vi "SERIAL_DecodeStreamResponse.vi"(8 "error in":errorcluster, 10 "Buffer":string, 11 "navX DevRef":T1={"SerialPortRef"={"DevStatus"={"status"=FALSE, "code"=0, "source"=""}, "Serial Port Name"=""}, "Board Information"={"WhoAmI (50 | 0x32)"=0, "Board Revision"=0, "Firmware Major Version"=0, "Firmware Minor Version"=0}, "Status"={"Update Rate Hz"=0, "Accelerometer Full-Scale Range"=0, "Gyro Full-Scale Range"=0, "NAVX_OP_STATUS"=0, "NAVX_CAL_STATUS"=0, "NAVX_SELFTEST_STATUS"=0, "NAVX_SENSOR_STATUS"=0}, "Offsets"={"Yaw"=0.0, "Quat W"=0.0, "Quat X"=0.0, "Quat Y"=0.0, "Quat Z"=0.0}, "Update Rate (4Hz-60Hz)"=50, "Nav6Mode (YPR)"=enum."YPR", "refnum name"="", "error"={"status"=FALSE, "code"=0, "source"=""}} {"Status"."NAVX_OP_STATUS" items=["INITIALIZING", "SELFTEST_IN_PROGRESS", "ERROR", "IMU_AUTOCAL_IN_PROGRESS", "NORMAL"]; "Status"."NAVX_CAL_STATUS" items=["IMU_CAL_STATE_MASK"=3, "IMU_CAL_INPROGRESS"=0, "IMU_CAL_ACCUMULATE"=1, "IMU_CAL_COMPLETE"=2, "MAG_CAL_COMPLETE"=4, "BARO_CAL_COMPLETE"=8]}) -> (0 "error out":errorcluster, 2 "Valid":bool, 3 "navX DevRef":T1={"SerialPortRef"={"DevStatus"={"status"=FALSE, "code"=0, "source"=""}, "Serial Port Name"=""}, "Board Information"={"WhoAmI (50 | 0x32)"=0, "Board Revision"=0, "Firmware Major Version"=0, "Firmware Minor Version"=0}, "Status"={"Update Rate Hz"=0, "Accelerometer Full-Scale Range"=0, "Gyro Full-Scale Range"=0, "NAVX_OP_STATUS"=0, "NAVX_CAL_STATUS"=0, "NAVX_SELFTEST_STATUS"=0, "NAVX_SENSOR_STATUS"=0}, "Offsets"={"Yaw"=0.0, "Quat W"=0.0, "Quat X"=0.0, "Quat Y"=0.0, "Quat Z"=0.0}, "Update Rate (4Hz-60Hz)"=50, "Nav6Mode (YPR)"=enum."YPR", "refnum name"="", "error"={"status"=FALSE, "code"=0, "source"=""}} {"Status"."NAVX_OP_STATUS" items=["INITIALIZING", "SELFTEST_IN_PROGRESS", "ERROR", "IMU_AUTOCAL_IN_PROGRESS", "NORMAL"]; "Status"."NAVX_CAL_STATUS" items=["IMU_CAL_STATE_MASK"=3, "IMU_CAL_INPROGRESS"=0, "IMU_CAL_ACCUMULATE"=1, "IMU_CAL_COMPLETE"=2, "MAG_CAL_COMPLETE"=4, "BARO_CAL_COMPLETE"=8]})   [LabVIEW 2014, in "navX-MXP IMU.lvlib"]
uses:
  navX-MXP IMU.lvlib
  navX Serial DevRef.ctl
  <vilib>/Rock Robotics/WPI/SerialPort/WPI_SerialPortRef.ctl
  COMMON/TypeDefs/navX Board Information.ctl
  COMMON/TypeDefs/navX Status Data.ctl
  COMMON/TypeDefs/navX NAVX_OP_STATUS.ctl
  COMMON/TypeDefs/navX NAVX_CAL_STATUS.ctl
  TypeDefs/navX Serial Mode.ctl
  COMMON/TypeDefs/navX Offsets Data.ctl
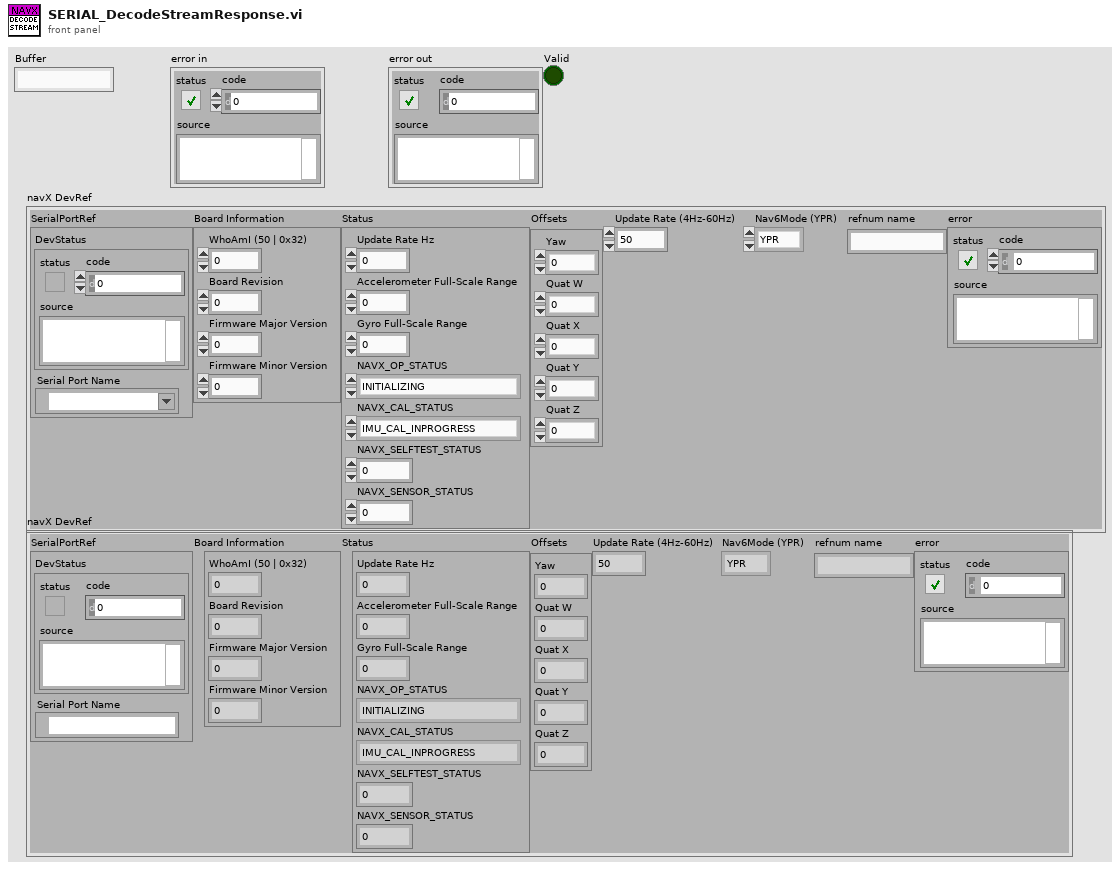
[diagram p1: front panel]
types:
  T1 = typedef "navX-MXP IMU.lvlib/navX Serial DevRef.ctl" = cluster{"SerialPortRef":T2, "Board Information":T3, "Status":T4, "Offsets":cluster{"Yaw":dbl, "Quat W":dbl, "Quat X":dbl, "Quat Y":dbl, "Quat Z":dbl}, "Update Rate (4Hz-60Hz)":u8, "Nav6Mode (YPR)":T7, "refnum name":string, "error":errorcluster}
  T2 = typedef "WPI_SerialPortRef.ctl" = cluster{"DevStatus":errorcluster, "Serial Port Name":refnum<visa-resource-name>}
  T3 = typedef "navX-MXP IMU.lvlib/navX Board Information.ctl" = cluster{"WhoAmI (50 | 0x32)":u8, "Board Revision":u8, "Firmware Major Version":u8, "Firmware Minor Version":u8}
  T4 = typedef "navX-MXP IMU.lvlib/navX Status Data.ctl" = cluster{"Update Rate Hz":u8, "Accelerometer Full-Scale Range":u8, "Gyro Full-Scale Range":u16, "NAVX_OP_STATUS":T5, "NAVX_CAL_STATUS":T6, "NAVX_SELFTEST_STATUS":u8, "NAVX_SENSOR_STATUS":u16}
  T5 = typedef "navX-MXP IMU.lvlib/navX NAVX_OP_STATUS.ctl" = u8
  T6 = typedef "navX-MXP IMU.lvlib/navX NAVX_CAL_STATUS.ctl" = u8
  T7 = typedef "navX-MXP IMU.lvlib/navX Serial Mode.ctl" = enum16{"YPR", "Gyro", "Quaternion"}
  T8 = typedef "navX-MXP IMU.lvlib/navX Offsets Data.ctl" = cluster{"Yaw":dbl, "Quat W":dbl, "Quat X":dbl, "Quat Y":dbl, "Quat Z":dbl}
  T9 = cluster{"Gyroscope Full Scale Range":u32, "Accelerometer Full Scale Range":u32, "Update Rate":u32, "Calibrated Yaw Offset":dbl, "Calibrated Quaternion W Offset ":u32, "Calibrated Quaternion X Offset":u32, "Calibrated Quaternion Y Offset":u32, "Calibrated Quaternion Z Offset":u32, "Flags":u32}
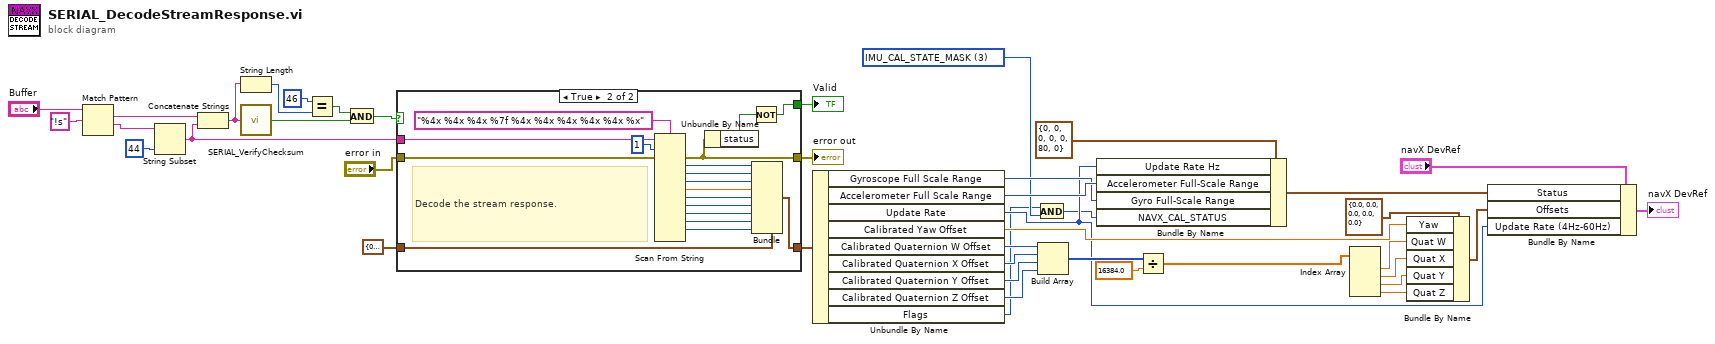
[diagram p0: block diagram]
diagram:
  w3 = T6 3 items=["IMU_CAL_STATE_MASK"=3, "IMU_CAL_INPROGRESS"=0, "IMU_CAL_ACCUMULATE"=1, "IMU_CAL_COMPLETE"=2, "MAG_CAL_COMPLETE"=4, "BARO_CAL_COMPLETE"=8] ("NAVX_CAL_STATUS")
  n1 = Match Pattern(string="Buffer", regular expression="!s") -> (match substring=w37:string, after substring=w39:string)  [unwired: 1 in, 2 out]
  n2 = String Subset(string=w39, length (rest)=44 ("length (rest)")) -> (substring=w26:string)  [unwired: 1 in]
  n3 = Concatenate Strings(w37, w26) -> (w27:string)
  n4 = String Length(string=w27) -> (length=w33:i32)
  n5 = call "SERIAL_VerifyChecksum.vi"("Content"=w27) -> ("Valid Checksum"=w36:bool)
  n6 = Equal?(x=46, y=w33) -> (x = y?=w31:bool)
  n7 = And(x=w31, y=w36) -> (x .and. y?=w35:bool)
  n8 = case shown="True" w35 {
    selector: w35 -> [w42 _]
    tunnel: [w43 w47] -> w34
    tunnel: w26 -> [_ w62]
    tunnel: [w44 w51] -> w25
    tunnel: T9 {"Gyroscope Full Scale Range"=0, "Accelerometer Full Scale Range"=0, "Update Rate"=0, "Calibrated Yaw Offset"=0.0, "Calibrated Quaternion W Offset "=0, "Calibrated Quaternion X Offset"=0, "Calibrated Quaternion Y Offset"=0, "Calibrated Quaternion Z Offset"=0, "Flags"=0} -> [w44 w50]
    tunnel: "error in" -> [w43 w49]
    tunnel: [w42 w45] -> w28
    frame False {
    }
    frame True {
      # "Decode the stream response."
      n9 = Scan From String(format string="%4x %4x %4x %7f %4x %4x %4x %4x %4x %x", input string=w62, initial scan location=u32 1, error in=w49) -> (error out=w47:errorcluster, output 1=w60:u32, output 2=w59:u32, output 3=w58:u32, output 4=w57:dbl, output 5=w56:u32, output 6=w55:u32, output 7=w54:u32, output 8=w53:u32, output 9=w52:u32)  [unwired: 11 in, 2 out]
      n10 = Unbundle By Name(w47) -> ("status"=w46:bool)
      n11 = Not(x=w46) -> (.not. x?=w45:bool)
      n12 = Bundle(cluster=w50, "Gyroscope Full Scale Range"=w60, "Accelerometer Full Scale Range"=w59, "Update Rate"=w58, "Calibrated Yaw Offset"=w57, "Calibrated Quaternion W Offset"=w56, "Calibrated Quaternion X Offset"=w55, "Calibrated Quaternion Y Offset"=w54, "Calibrated Quaternion Z Offset"=w53, "Flags"=w52) -> (w51:T9)
    }
  }
  "error out" <- w34
  "Valid" <- w28
  n13 = Unbundle By Name(w25) -> ("Gyroscope Full Scale Range"=w22:u32, "Accelerometer Full Scale Range"=w23:u32, "Update Rate"=w4:u32, "Calibrated Yaw Offset"=w21:dbl, "Calibrated Quaternion W Offset"=w20:u32, "Calibrated Quaternion X Offset"=w17:u32, "Calibrated Quaternion Y Offset"=w18:u32, "Calibrated Quaternion Z Offset"=w19:u32, "Flags"=w2:u32)
  n14 = And(x=w2, y=w3) -> (x .and. y?=w1:u32)
  n15 = Build Array(w20, w17, w18, w19) -> (w15:u32[])
  n16 = Bundle By Name(cluster=T4 {"Update Rate Hz"=0, "Accelerometer Full-Scale Range"=0, "Gyro Full-Scale Range"=0, "NAVX_OP_STATUS"=0, "NAVX_CAL_STATUS"=0, "NAVX_SELFTEST_STATUS"=80, "NAVX_SENSOR_STATUS"=0} ("Status"), "Update Rate Hz"=w4, "Accelerometer Full-Scale Range"=w23, "Gyro Full-Scale Range"=w22, "NAVX_CAL_STATUS"=w1) -> (w7:T4)
  n17 = Divide(x=w15, y=16384.0) -> (x/y=w14:dbl[])
  n18 = Index Array(array=w14) -> (element #1=w13:dbl, element #2=w12:dbl, element #3=w11:dbl, element #4=w10:dbl)  [unwired: 4 in]
  n19 = Bundle By Name(cluster=T8 {"Yaw"=0.0, "Quat W"=0.0, "Quat X"=0.0, "Quat Y"=0.0, "Quat Z"=0.0} ("Offsets"), "Yaw"=w21, "Quat W"=w13, "Quat X"=w12, "Quat Y"=w11, "Quat Z"=w10) -> (w5:T8)
  n20 = Bundle By Name(cluster="navX DevRef", "Status"=w7, "Offsets"=w5, "Update Rate (4Hz-60Hz)"=w4) -> (→"navX DevRef":T1)
